vi "7. Add Label.vi"(6 "Variant in":variant, 7 "Shift Pressed?":bool, 8 "error in (no error)":errorcluster, 10 "QD Combo Box Ref":refnum<vi>, 11 "QD Launch VI Ref":refnum<vi>) -> (0 "error out":errorcluster, 4 "Variant out":variant)   [LabVIEW 2012]
doc: "Default Shortcut - [7]"
uses:
  <vilib>/Utility/config.llb/Read Key (String).vi
  <vilib>/Utility/config.llb/NI_LVConfig.lvlib
panel:
  in  "Undo Name":string="Quick Drop Keyboard Shortcut"
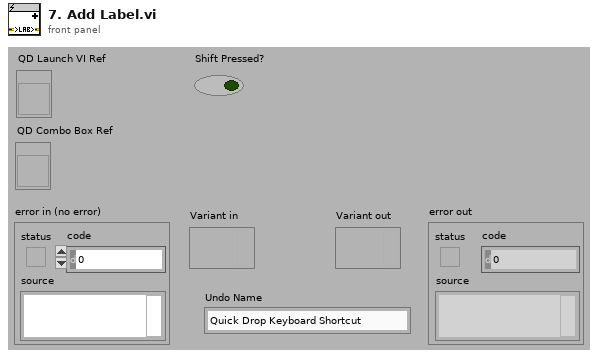
[diagram p1: front panel]
types:
  T1 = typedef "NI_LVConfig.lvlib/Config Data RefNum.ctl" = refnum<k1>
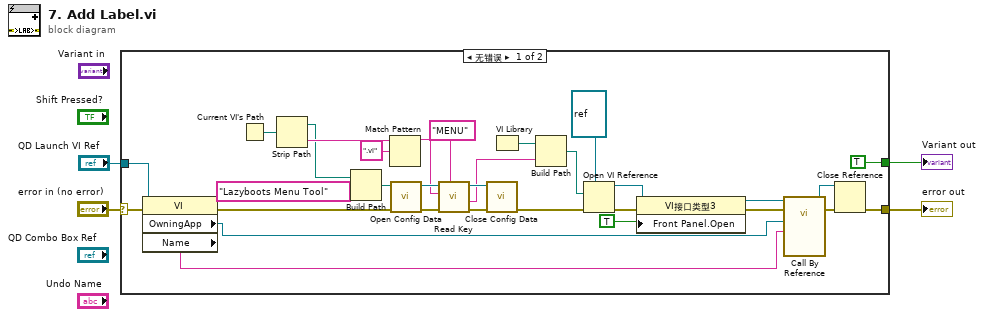
[diagram p0: block diagram]
diagram:
  n1 = case shown="无错误" "error in (no error)" {
    selector: "error in (no error)" -> [w35 w36]
    tunnel: [w34 w36] -> w3
    tunnel: "QD Launch VI Ref" -> [w33 _]
    tunnel: [TRUE _] -> w1
    frame No Error {
      n2 = property class="VI"(reference=w33, error in=w35) -> (error out=w12:errorcluster, "OwningApp"=w14:refnum<vi>, "Name"=w13:string)  [unwired: 1 out]
      n3 = Current VI's Path() -> (path=w28:path)
      n4 = Strip Path(path=w28) -> (stripped path=w10:path, name=w20:string)
      n5 = Build Path(base path=w10, name or relative path="Lazyboots Menu Tool") -> (appended path=w26:path)
      n6 = Match Pattern(string=w20, regular expression=".vi") -> (before substring=w19:string)  [unwired: 4 out]
      n7 = call <vilib>:"Open Config Data.vi"("error in (no error)"=w12, "configuration file path"=w26) -> ("error out"=w24:errorcluster, "refnum"=w25:T1)  [unwired: 7 in, 1 out]
      n8 = call-poly <vilib>:"Read Key.vi"("section"="MENU", "error in (no error)"=w24, "key"=w19, "refnum"=w25) -> ("error out"=w21:errorcluster, "value"=w16:string, "refnum out"=w22:T1)  [unwired: 2 in, 3 out]
      n9 = call <vilib>:"Close Config Data.vi"("error in (no error)"=w21, "refnum"=w22) -> ("error out"=w11:errorcluster)  [unwired: 1 in, 8 out]
      n10 = VI Library() -> (path=w15:path)
      n11 = Build Path(base path=w15, name or relative path=w16) -> (appended path=w17:path)
      n12 = Open VI Reference(type specifier VI Refnum (for type only)=refnum<vi> refnum, vi path=w17, error in (no error)=w11) -> (vi reference=w7:refnum<vi>, error out=w30:errorcluster)  [unwired: 3 out]
      n13 = property class="VI接口类型3"(reference=w7, error in=w30, "Front Panel.Open"=TRUE ("Front Panel Window:Open")) -> (reference out=w6:refnum<vi>, error out=w8:errorcluster)
      n14 = call-by-ref "?"(reference=w6, error in=w8, "VI Path"=w13, "Application Reference"=w14) -> (reference out=w9:refnum<vi>, error out=w29:errorcluster)  [unwired: 9 in, 1 out]
      n15 = Close Reference(reference=w9, error in (no error)=w29) -> (error out=w34:errorcluster)
    }
    frame Error {
    }
  }
  "error out" <- w3
  "Variant out" <- w1
